vi "plot_display.vi"(0 "Input Graph Data":cluster{dbl[], dbl[]}(graph), 1 "X Scale.Name Label.Text":string, 2 "Y Scale.Name Label.Text":string, 3 "FileName":string, 6 "xValues":i32, 8 "yValues":i32, 10 "File Path":path) -> ()   [LabVIEW 2019]
uses:
  <vilib>/Utility/miscctls.llb/LVForegroundBackgroundColorsTypeDef.ctl
  <vilib>/Analysis/Matrix/Numeric/Conversions/Array To Matrix - RA2.vi
  <vilib>/Analysis/Matrix/Numeric/Conversions/Matrix To Array - RM.vi
  <vilib>/Analysis/Matrix/NI_Matrix.lvlib
panel:
  out "XY-Graph":cluster{dbl[], dbl[]}(graph)
  in  "OK Button":bool
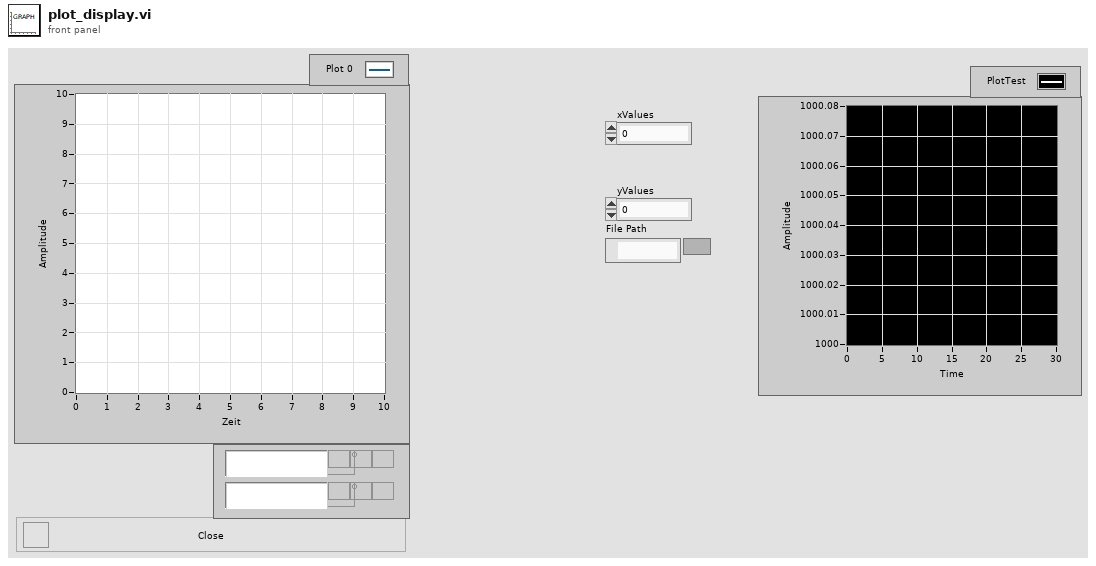
[diagram p1: front panel]
types:
  T1 = typedef "LVForegroundBackgroundColorsTypeDef.ctl" = cluster{"Foreground Color":u32, "Background Color":u32}
  T2 = enum32{"Invalid", "Standard", "Closed", "Hidden", "Minimized", "Maximized"}
  T3 = typedef "NI_Matrix.lvlib/RealMatrix.ctl" = dbl[][]
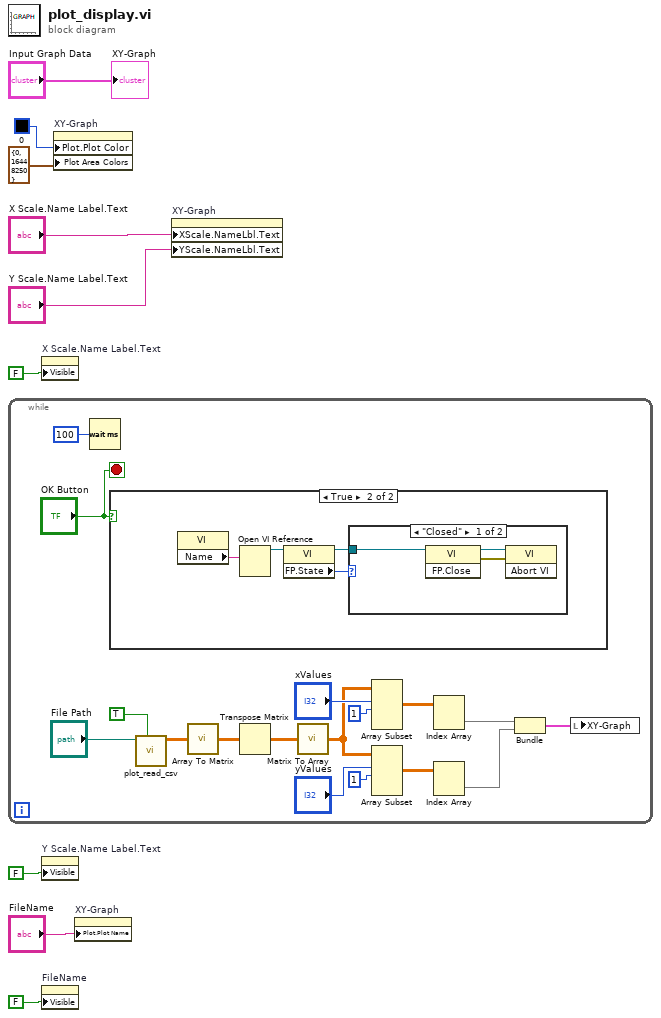
[diagram p0: block diagram]
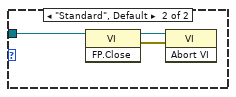
[diagram p3: hidden frame]
diagram:
  n1 = while {
    stop <- "OK Button" stop-if-true
    n2 = Wait (ms)(milliseconds to wait=u32 100) -> ()  [unwired: 1 out]
    n3 = case shown="True" "OK Button" {
      frame False {
      }
      frame True {
        n4 = property class="VI"() -> ("Name"=w30:string)  [unwired: 2 in, 2 out]
        n5 = Open VI Reference(vi path=w30) -> (vi reference=w29:refnum<vi>)  [unwired: 5 in, 1 out]
        n6 = property class="VI"(reference=w29) -> (reference out=w27:refnum<vi>, "FP.State"=w28:T2)  [unwired: 1 in, 1 out]
        n7 = case shown="\"Closed\"" w28 {
          tunnel: w27 -> [w31 w36]
          frame "Closed" {
            n8 = invoke class="VI" method="FP.Close"(reference=w31) -> (reference out=w33:refnum<vi>, error out=w32:errorcluster)  [unwired: 2 in, 1 out]
            n9 = invoke class="VI" method="Abort VI"(reference=w33, error in=w32) -> ()  [unwired: 1 in, 3 out]
          }
          frame "Standard", Default {
            n10 = invoke class="VI" method="FP.Close"(reference=w36) -> (reference out=w35:refnum<vi>, error out=w34:errorcluster)  [unwired: 2 in, 1 out]
            n11 = invoke class="VI" method="Abort VI"(reference=w35, error in=w34) -> ()  [unwired: 1 in, 3 out]
          }
        }
      }
    }
    n12 = call "plot_read_csv.vi"("Read"=TRUE, "Read File:"="File Path") -> ("File Data"=w16:T3)  [unwired: 9 in]
    n13 = call-poly <vilib>:"Array To Matrix.vi"("Real 2D Array"=w16) -> ("Real Matrix"=w25:T3)
    n14 = Transpose Matrix(1:w25) -> (0:w26:T3)
    n15 = call-poly <vilib>:"Matrix To Array.vi"("Real Matrix"=w26) -> ("Real 2D Array"=w22:dbl[][])
    n16 = Array Subset(array=w22, index (row)="xValues", length (row)=1 ("length")) -> (w21:dbl[][])  [unwired: 2 in]
    n17 = Array Subset(array=w22, index (row)="yValues", length (row)=1 ("length")) -> (w19:dbl[][])  [unwired: 2 in]
    n18 = Index Array(array=w21) -> (element=w20:dbl[])  [unwired: 2 in]
    n19 = Index Array(array=w19) -> (element=w18:dbl[])  [unwired: 2 in]
    n20 = Bundle(w20, w18) -> (w10:cluster{dbl[], dbl[]})  [unwired: 1 in]
    n21 = local write "XY-Graph"(w10) -> ()
  }
  n22 = property on="X Scale.Name Label.Text" class="Str"("Visible"=FALSE) -> ()  [unwired: 2 in, 2 out]
  n23 = property on="Y Scale.Name Label.Text" class="Str"("Visible"=FALSE) -> ()  [unwired: 2 in, 2 out]
  n24 = property on="FileName" class="Str"("Visible"=FALSE) -> ()  [unwired: 2 in, 2 out]
  n25 = property on="XY-Graph" class="XYGraph (strict)"("Plot.Plot Color"=u32 0, "Plot Area Colors"=T1 {"Foreground Color"=0, "Background Color"=16448250} ("Plot Area:Colors")) -> ()  [unwired: 2 in, 2 out]
  n26 = property on="XY-Graph" class="XYGraph (strict)"("Plot.Plot Name"="FileName") -> ()  [unwired: 2 in, 2 out]
  n27 = property on="XY-Graph" class="XYGraph (strict)"("XScale.NameLbl.Text"="X Scale.Name Label.Text", "YScale.NameLbl.Text"="Y Scale.Name Label.Text") -> ()  [unwired: 2 in, 2 out]
  "XY-Graph" <- "Input Graph Data"
